vi "DAQmx Advance Trigger (None).vi"(0 "task/channels in":refnum<k21>, 11 "error in":errorcluster) -> (4 "task out":refnum<k21>, 15 "error out":errorcluster)   [LabVIEW 2011]
doc: "Disables advance triggering for the task."
uses:
  C:/Program Files/National Instruments/LabVIEW 2011/resource/objmgr/daqmx.rc
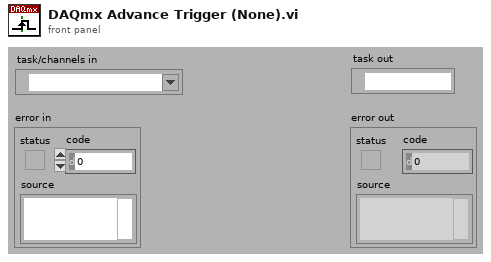
[diagram p1: front panel]
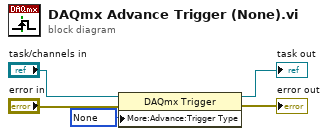
[diagram p0: block diagram]
diagram:
  w1 = 10230 items=["Digital Edge"=10150, "Software"=10292, "None"=10230] ("Adv.TrigType")
  n1 = property class="DAQmx Trigger"(reference="task/channels in", error in="error in", "More:Advance:Trigger Type"=w1) -> (reference out=→"task out":refnum<k21>, error out=→"error out":errorcluster)
